vi "Variant to Datatype.vi"(4 "Variant":variant) -> (0 "Value":string, 1 "Name":string, 2 "Datatype":T1)   [LabVIEW 2016]
uses:
  Datatype.ctl
  <userlib>/_OpenG.lib/lvdata/lvdata.llb/Type Descriptor Enumeration__ogtk.ctl
  <vilib>/Utility/Data Type/NI_Data Type.lvlib
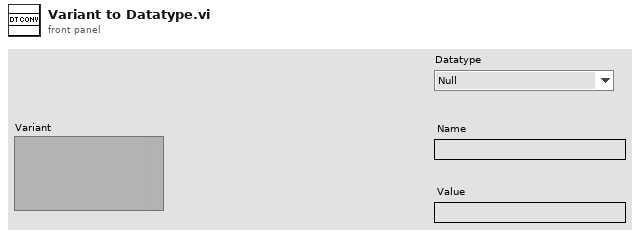
[diagram p1: front panel]
types:
  T1 = typedef "Datatype.ctl" = enum16{"Null", "Numeric", "String", "Bool", "Numeric 1D", "String 1D", "Bool 1D", "Numeric 2D", "String 2D", "Bool 2D", "Variant"}
  T2 = typedef "Type Descriptor Enumeration__ogtk.ctl" = enum8{"<Null>", "I8", "I16", "I32", "I64", "U8", "U16", "U32", "U64", "SGL", "DBL", "EXT", "CSG", "CDB", "CXT", "0x0F", "0x10", "0x11", "0x12", "0x13", "0x14", "Enum U8", "Enum U16", "Enum U32", "Enum U64", "SGL PQ", "DBL PQ", "EXT PQ", "CSG PQ", "CDB PQ", "CXT PQ", "0x1F", "0x20", "Boolean", "0x22", "0x23", "0x24", "0x25", "0x26", "0x27", "0x28", "0x29", "0x2A", "0x2B", "0x2C", "0x2D", "0x2E", "0x2F", "String", "0x31", "Path", "Pict", "0x34", "0x35", "0x36", "DAQ", "0x38", "0x39", "0x3A", "0x3B", "0x3C", "0x3D", "0x3E", "0x3F", "Array", "0x41", "0x42", "0x43", "0x44", "0x45", "0x46", "0x47", "0x48", "0x49", "0x4A", "0x4B", "0x4C", "0x4D", "0x4E", "0x4F", "Cluster", "0x51", "0x52", "Variant", "Waveform", "0x55", "0x56", "0x57", "0x58", "0x59", "0x5A", "0x5B", "0x5C", "0x5D", "0x5E", "0x5F", "0x60", "0x61", "0x62", "0x63", "0x64", "0x65", "0x66", "0x67", "0x68", "0x69", "0x6A", "0x6B", "0x6C", "0x6D", "0x6E", "0x6F", "Refnum"}
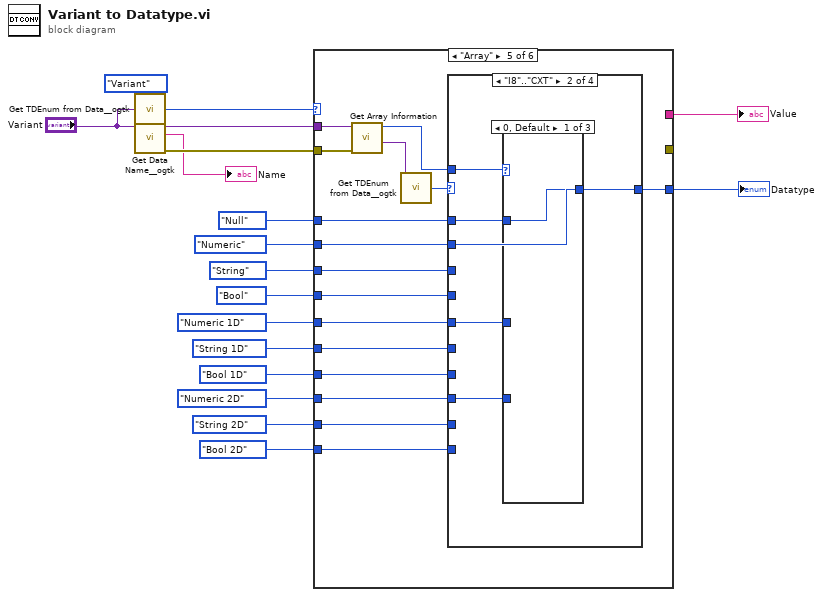
[diagram p0: block diagram]
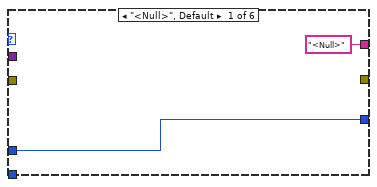
[diagram p2: hidden frame]
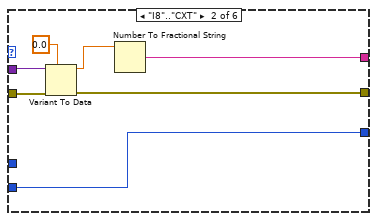
[diagram p3: hidden frame]
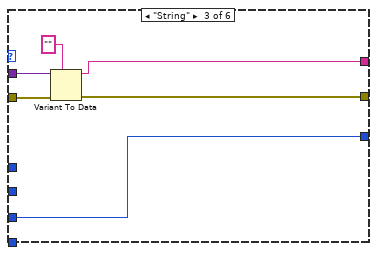
[diagram p4: hidden frame]
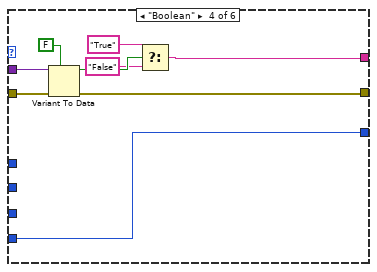
[diagram p5: hidden frame]
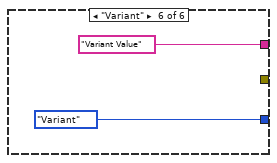
[diagram p15: hidden frame]
diagram:
  (unwired) Type_Descriptor_Enumeration__ogtk."Variant" ("Type Descriptor Enumeration")
  n1 = call <userlib>:"Get TDEnum from Data__ogtk.vi"("Data"="Variant") -> ("Type Descriptor Enumeration"=w11:T2)  [unwired: 4 in]
  n2 = call <userlib>:"Get Data Name__ogtk.vi"("Data"="Variant") -> ("error out"=w10:errorcluster, "Data Name"=→"Name":string, "Data dup"=w8:variant)  [unwired: 8 in]
  n3 = case shown="\"Array\"" w11 {
    tunnel: [w19 w26 w32 w41 w53 Datatype."Variant" ("Datatype")] -> w17
    tunnel: Datatype."Null" ("Datatype") -> [w19 _ _ _ w52 _]
    tunnel: Datatype."Numeric" ("Datatype") -> [_ w26 _ _ w51 _]
    tunnel: Datatype."String" ("Datatype") -> [_ _ w32 _ w50 _]
    tunnel: Datatype."Bool" ("Datatype") -> [_ _ _ w41 w49 _]
    tunnel: w10 -> [_ w24 w29 w38 w56 _]
    tunnel: w8 -> [_ w25 w30 w39 w57 _]
    tunnel: Datatype."Numeric 1D" ("Datatype") -> [_ _ _ _ w48 _]
    tunnel: Datatype."String 1D" ("Datatype") -> [_ _ _ _ w47 _]
    tunnel: Datatype."Bool 1D" ("Datatype") -> [_ _ _ _ w46 _]
    tunnel: Datatype."Numeric 2D" ("Datatype") -> [_ _ _ _ w45 _]
    tunnel: Datatype."String 2D" ("Datatype") -> [_ _ _ _ w44 _]
    tunnel: Datatype."Bool 2D" ("Datatype") -> [_ _ _ _ w43 _]
    tunnel: ["<Null>" w21 w28 w35 _ "Variant Value"] -> w1
    tunnel: [_ w20 w27 w37 _ _] -> _
    frame "<Null>", Default {
    }
    frame "I8".."CXT" {
      n4 = Variant To Data(error in=w24, type=0.0, Variant=w25) -> (data=w22:dbl, error out=w20:errorcluster)
      n5 = Number To Fractional String(number=w22) -> (F-format string=w21:string)  [unwired: 3 in]
    }
    frame "String" {
      n6 = Variant To Data(error in=w29, type="", Variant=w30) -> (data=w28:string, error out=w27:errorcluster)
    }
    frame "Boolean" {
      n7 = Variant To Data(error in=w38, type=FALSE, Variant=w39) -> (data=w36:bool, error out=w37:errorcluster)
      n8 = Select(t="True", s=w36, f="False") -> (s? t:f=w35:string)
    }
    frame "Array" {
      n9 = call <vilib>:"Get Array Information.vi"("error in (no error)"=w56, "Variant"=w57) -> ("Array Element Data Type"=w55:variant, "Number of Dimensions"=w42:i32)  [unwired: 6 in, 2 out]
      n10 = call <userlib>:"Get TDEnum from Data__ogtk.vi"("Data"=w55) -> ("Type Descriptor Enumeration"=w54:T2)  [unwired: 4 in]
      n11 = case shown="\"I8\"..\"CXT\"" w54 {
        tunnel: [w58 w63 w71 w78] -> w53
        tunnel: w52 -> [w58 w61 w70 w77]
        tunnel: w51 -> [_ w63 _ _]
        tunnel: w50 -> [_ _ w71 _]
        tunnel: w49 -> [_ _ _ _]
        tunnel: w48 -> [_ w60 _ _]
        tunnel: w47 -> [_ _ w68 _]
        tunnel: w46 -> [_ _ _ w76]
        tunnel: w45 -> [_ w59 _ _]
        tunnel: w44 -> [_ _ w67 _]
        tunnel: w43 -> [_ _ _ w75]
        tunnel: w42 -> [_ w62 w69 w79]
        frame "<Null>", Default {
        }
        frame "I8".."CXT" {
          n12 = case shown="0, Default" w62 {
            tunnel: [w64 w65 w66] -> _
            tunnel: w61 -> [w64 _ _]
            tunnel: w60 -> [_ w65 _]
            tunnel: w59 -> [_ _ w66]
            frame 0, Default {
            }
            frame 1 {
            }
            frame 2 {
            }
          }
        }
        frame "String" {
          n13 = case shown="2" w69 {
            tunnel: [w72 w73 w74] -> _
            tunnel: w70 -> [w72 _ _]
            tunnel: w68 -> [_ w73 _]
            tunnel: w67 -> [_ _ w74]
            frame 0, Default {
            }
            frame 1 {
            }
            frame 2 {
            }
          }
        }
        frame "Boolean" {
          n14 = case shown="2" w79 {
            tunnel: [w80 w81 w82] -> w78
            tunnel: w77 -> [w80 _ _]
            tunnel: w76 -> [_ w81 _]
            tunnel: w75 -> [_ _ w82]
            frame 0, Default {
            }
            frame 1 {
            }
            frame 2 {
            }
          }
        }
      }
    }
    frame "Variant" {
    }
  }
  "Datatype" <- w17
  "Value" <- w1
